vi "DeleteData.vi"(8 "error in (no error)":errorcluster caption="entrée d'erreur (pas d'erreur)", 10 "CurveNumber":i32, 11 "Interface en entrée":refnum<class "Interface.lvclass"> caption="DNL_LabVIEW Object in") -> (0 "error out":errorcluster caption="sortie d'erreur", 3 "Interface en sortie":refnum<class "Interface.lvclass"> caption="DNL_LabVIEW Object out")   [LabVIEW 2019, in "Interface.lvclass"]
uses:
  Interface.lvclass
  Interface.lvclass/Interface.ctl
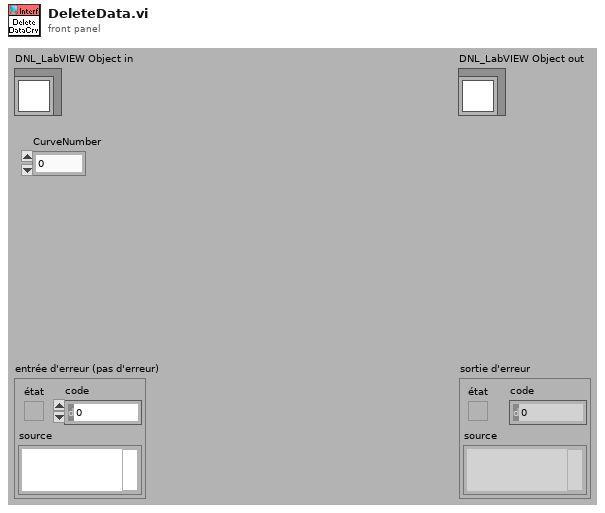
[diagram p1: front panel]
types:
  T1 = typedef "Interface.lvclass/CurveSetup.ctl" = cluster{"CurveName":string, "YParam":string, "XParam":string, "ZParam ":string, "GroupName":string, "LinWdth":u8, "PntCol":u32, "LinCol":u32, "LablFor":u8, "XScale":u32, "YScale":u32, "Interpol":u8, "DisplayName":string, "FillType":i16, "LineStyle":u8, "PntStyle":u8, "BarTyp":u8, "GraphIndex":i32, "Visible":bool, "XScaleName":string, "YScaleName":string, "XYGraph_Ref":refnum<vi>, "Data Only":bool, "DataQ Ref":refnum<queue>, "XParQ Ref":refnum<queue>, "XParamInd":i32, "ScanInd":i32, "File Path":path}
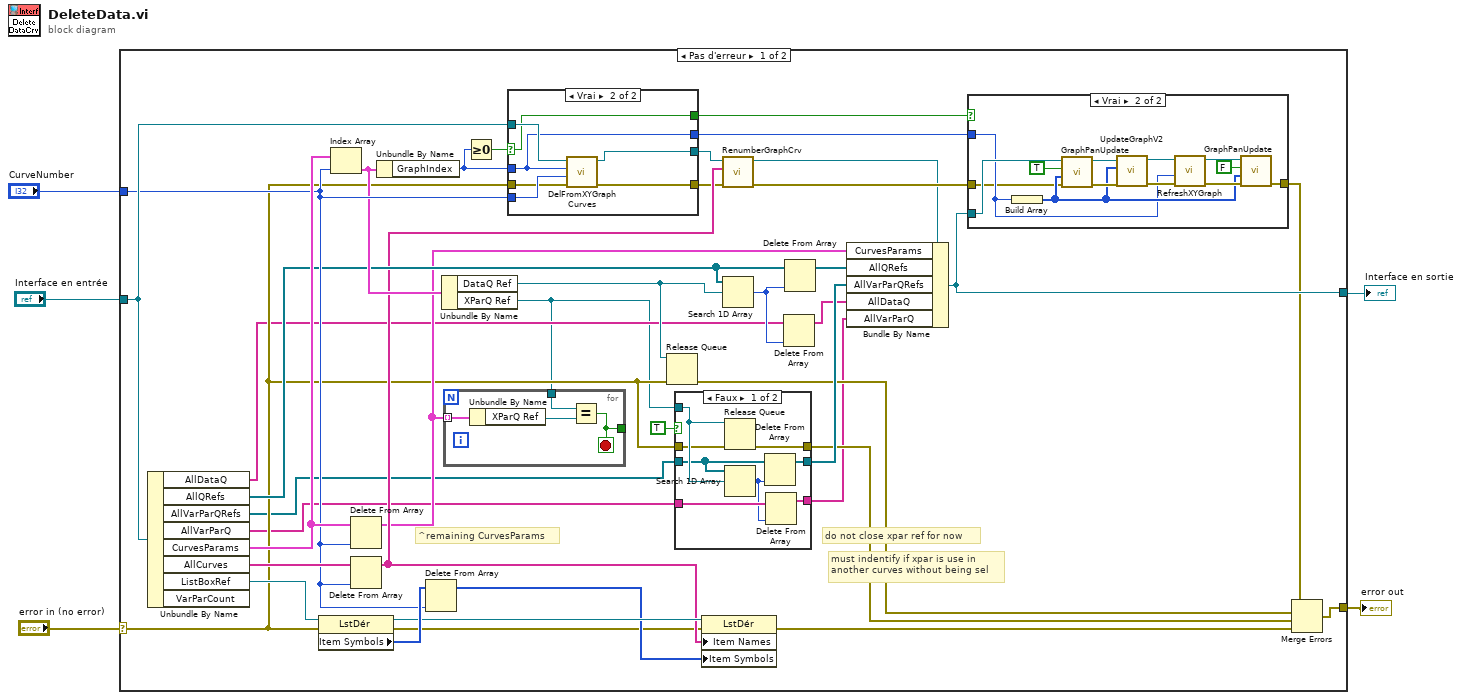
[diagram p0: block diagram]
diagram:
  n1 = case shown="Pas d'erreur" "error in (no error)" {
    selector: "error in (no error)" -> [w28 w86]
    tunnel: [w22 w86] -> w4
    tunnel: [w25 w85] -> w2
    tunnel: "Interface en entrée" -> [w43 w85]
    tunnel: "CurveNumber" -> [w38 _]
    frame No Error {
      # "do not close xpar ref for now"
      # "must indentify if xpar is use in\nanother curves without being sel"
      # "^remaining CurvesParams"
      n2 = Unbundle By Name(w43) -> ("AllDataQ"=w16:string[], "AllQRefs"=w34:refnum<queue>[], "AllVarParQRefs"=w14:refnum<queue>[], "AllVarParQ"=w13:string[], "CurvesParams"=w40:T1[], "AllCurves"=w41:string[], "ListBoxRef"=w42:refnum<vi>)  [unwired: 1 out]
      n3 = property class="LstDér"(reference=w42, error in=w28) -> (reference out=w37:refnum<vi>, error out=w29:errorcluster, "Item Symbols"=w39:i32[])
      n4 = Index Array(array=w40, index=w38) -> (element=w35:T1)
      n5 = Delete From Array(array=w40, index=w38) -> (array with subset deleted=w31:T1[])  [unwired: 1 in, 1 out]
      n6 = Delete From Array(array=w41, index=w38) -> (array with subset deleted=w32:string[])  [unwired: 1 in, 1 out]
      n7 = Unbundle By Name(w35) -> ("GraphIndex"=w44:i32)
      n8 = Delete From Array(array=w39, index=w38) -> (array with subset deleted=w36:i32[])  [unwired: 1 in, 1 out]
      n9 = Unbundle By Name(w35) -> ("DataQ Ref"=w33:refnum<queue>, "XParQ Ref"=w7:refnum<queue>)
      n10 = for {
        tunnel: w31 -> [w73] mode=indexing
        tunnel: w7 -> [w72]
        tunnel: [w70] -> _
        stop <- w70 stop-if-true
        n11 = Unbundle By Name(w73) -> ("XParQ Ref"=w71:refnum<queue>)
        n12 = Equal?(x=w72, y=w71) -> (x = y?=w70:bool)
      }
      n13 = Greater Or Equal To 0?(x=w44) -> (x >= 0?=w26:bool)
      n14 = case shown="Vrai" w26 {
        selector: w26 -> [w76 w80]
        tunnel: w38 -> [_ w83]
        tunnel: w44 -> [w75 w81]
        tunnel: w43 -> [w74 w84]
        tunnel: w28 -> [w77 w82]
        tunnel: [w77 w78] -> w8
        tunnel: [w75 w81] -> w23
        tunnel: [w76 w80] -> w24
        tunnel: [w74 w79] -> w11
        frame False {
          # "curves was not graphed"
        }
        frame True {
          n15 = call "DelFromXYGraphCurves.vi"("error in (no error)"=w82, "CurvIndex"=w83, "GraphIndex"=w81, "Interface en entrée"=w84) -> ("error out"=w78:errorcluster, "Interface en sortie"=w79:refnum<class "Interface.lvclass">)  [unwired: 6 in]
        }
      }
      n16 = Release Queue(queue=w33, error in (no error)=w28) -> (error out=w20:errorcluster)  [unwired: 1 in, 2 out]
      n17 = case shown="Faux" TRUE {
        tunnel: w7 -> [w66 _]
        tunnel: w14 -> [w65 w69]
        tunnel: [w64 w69] -> w27
        tunnel: w28 -> [w63 w68]
        tunnel: [w62 w68] -> w19
        tunnel: w13 -> [w61 w67]
        tunnel: [w59 w67] -> w12
        frame False {
          n18 = Release Queue(queue=w66, error in (no error)=w63) -> (error out=w62:errorcluster)  [unwired: 1 in, 2 out]
          n19 = Search 1D Array(1D array=w65, element=w66) -> (index of element=w60:i32)  [unwired: 1 in]
          n20 = Delete From Array(array=w65, index=w60) -> (array with subset deleted=w64:refnum<queue>[])  [unwired: 1 in, 1 out]
          n21 = Delete From Array(array=w61, index=w60) -> (array with subset deleted=w59:string[])  [unwired: 1 in, 1 out]
        }
        frame True {
          # "there are still crvsusing that q!"
        }
      }
      n22 = property class="LstDér"(reference=w37, error in=w29, "Item Names"=w32, "Item Symbols"=w36) -> (error out=w18:errorcluster)  [unwired: 1 out]
      n23 = call "RenumberGraphCrv.vi"("error in (no error)"=w8, "AllCurves"=w32, "Interface en entrée"=w11) -> ("error out"=w10:errorcluster, "Interface en sortie"=w9:refnum<class "Interface.lvclass">)  [unwired: 7 in]
      n24 = Search 1D Array(1D array=w34, element=w33) -> (index of element=w17:i32)  [unwired: 1 in]
      n25 = Delete From Array(array=w16, index=w17) -> (array with subset deleted=w15:string[])  [unwired: 1 in, 1 out]
      n26 = Delete From Array(array=w34, index=w17) -> (array with subset deleted=w30:refnum<queue>[])  [unwired: 1 in, 1 out]
      n27 = Bundle By Name(cluster=w9, "CurvesParams"=w31, "AllQRefs"=w30, "AllVarParQRefs"=w27, "AllDataQ"=w15, "AllVarParQ"=w12) -> (w25:refnum<class "Interface.lvclass">)
      n28 = case shown="Vrai" w24 {
        tunnel: w25 -> [_ w49]
        tunnel: w23 -> [_ w48]
        tunnel: w10 -> [w45 w47]
        tunnel: [w45 w46] -> w21
        frame False {
        }
        frame True {
          n29 = Build Array(w48) -> (w53:i32[])
          n30 = call "GraphPanUpdate.vi"("error in (no error)"=w47, "GraphInd"=w53, "DeferUpdate"=TRUE, "Interface en entrée"=w49) -> ("error out"=w58:errorcluster, "Interface en sortie"=w57:refnum<class "Interface.lvclass">)  [unwired: 6 in]
          n31 = call "UpdateGraphV2.vi"("error in (no error)"=w58, "GraphIndexArr"=w53, "Interface en entrée"=w57) -> ("error out"=w52:errorcluster, "Interface en sortie"=w55:refnum<class "Interface.lvclass">)  [unwired: 7 in]
          n32 = call "RefreshXYGraph.vi"("error in (no error)"=w52, "Graph Index"=w48, "Interface en entrée"=w55) -> ("error out"=w54:errorcluster, "Interface en sortie"=w56:refnum<class "Interface.lvclass">)  [unwired: 6 in, 1 out]
          n33 = call "GraphPanUpdate.vi"("error in (no error)"=w54, "GraphInd"=w53, "DeferUpdate"=FALSE, "Interface en entrée"=w56) -> ("error out"=w46:errorcluster)  [unwired: 6 in, 1 out]
        }
      }
      n34 = Merge Errors(w21, w20, w19, w18) -> (w22:errorcluster)
    }
    frame Error {
    }
  }
  "error out" <- w4
  "Interface en sortie" <- w2
